vi "读取开始接收数据？.vi"(8 "error in (no error)":errorcluster, 11 "串口通信类 in":refnum<class "串口通信类.lvclass">) -> (0 "error out":errorcluster, 2 "开始接收数据？":bool, 3 "串口通信类 out":refnum<class "串口通信类.lvclass">)   [LabVIEW 2015, in "串口通信类.lvclass"]
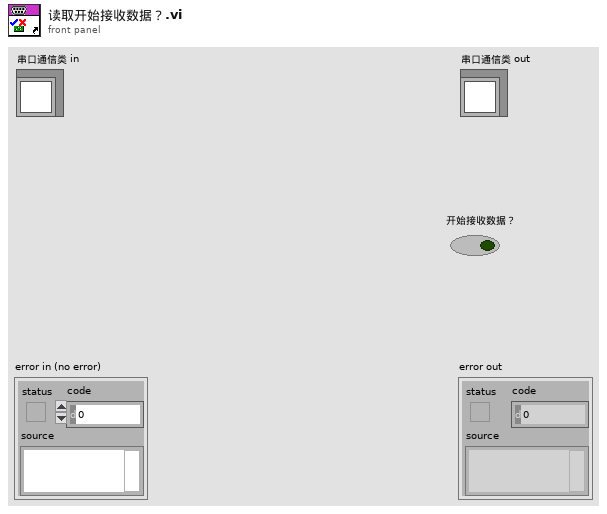
[diagram p1: front panel]
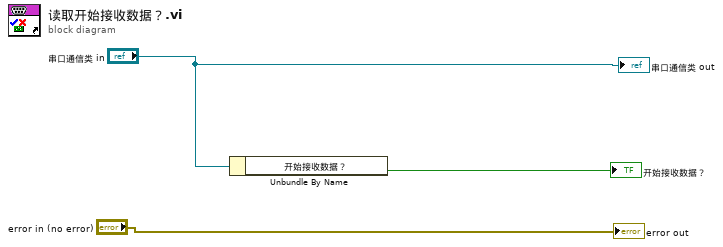
[diagram p0: block diagram]
diagram:
  n1 = Unbundle By Name("串口通信类 in") -> ("开始接收数据？"=→"开始接收数据？":bool)
  "error out" <- "error in (no error)"
  "串口通信类 out" <- "串口通信类 in"
